vi "DOE Water Temperature Pressure.vi"(5 "Water Pressure":dbl, 6 "Data Logger Type":T1=enum."Agilent", 7 "Water Temperature":dbl, 8 "Error In":errorcluster, 9 "Output Array":dbl[](array[numeric]), 10 "TC Coefficients":T2, 11 "Kitchen Cluster in":T3) -> (0 "Error Out":errorcluster, 3 "Kitchen Cluster out":T3, 4 "sorted array":i32[](array[numeric]))   [LabVIEW 2016]
uses:
  Type Definitions/DOE Kitchen Control.ctl
  Utility/Type Definitions/UTILITY TC Coefficients.ctl
  Type Definitions/DOE Data Logger Type.ctl
  Utility/Type Definitions/UTILITY TC Coefficients Selector.ctl
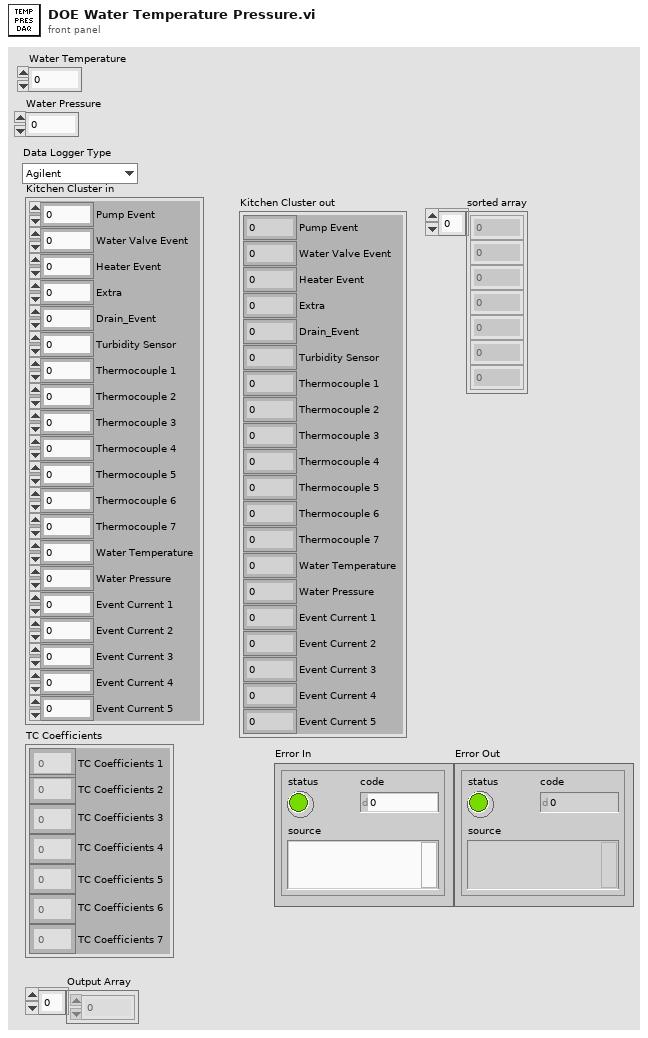
[diagram p1: front panel]
types:
  T1 = typedef "DOE Data Logger Type.ctl" = enum16{"MW100", "Agilent", "Agilent_Laurel_DC_Clamp"}
  T2 = typedef "UTILITY TC Coefficients.ctl" = cluster{"TC Coefficients 1":dbl[], "TC Coefficients 2":dbl[], "TC Coefficients 3":dbl[], "TC Coefficients 4":dbl[], "TC Coefficients 5":dbl[], "TC Coefficients 6":dbl[], "TC Coefficients 7":dbl[]}
  T3 = typedef "DOE Kitchen Control.ctl" = cluster{"Drain_Event":i16, "Pump Event":i16, "Water Valve Event":i16, "Heater Event":i16, "Extra":i16, "Turbidity Sensor":dbl, "Thermocouple 1":dbl, "Thermocouple 2":dbl, "Thermocouple 3":dbl, "Thermocouple 4":dbl, "Thermocouple 5":dbl, "Thermocouple 6":dbl, "Water Temperature":dbl, "Water Pressure":dbl, "Event Current 1":dbl, "Event Current 2":dbl, "Event Current 3":dbl, "Event Current 4":dbl, "Event Current 5":dbl, "Thermocouple 7":dbl}
  T4 = typedef "UTILITY TC Coefficients Selector.ctl" = enum16{"TC1", "TC2", "TC3", "TC4", "TC5", "TC6", "TC7"}
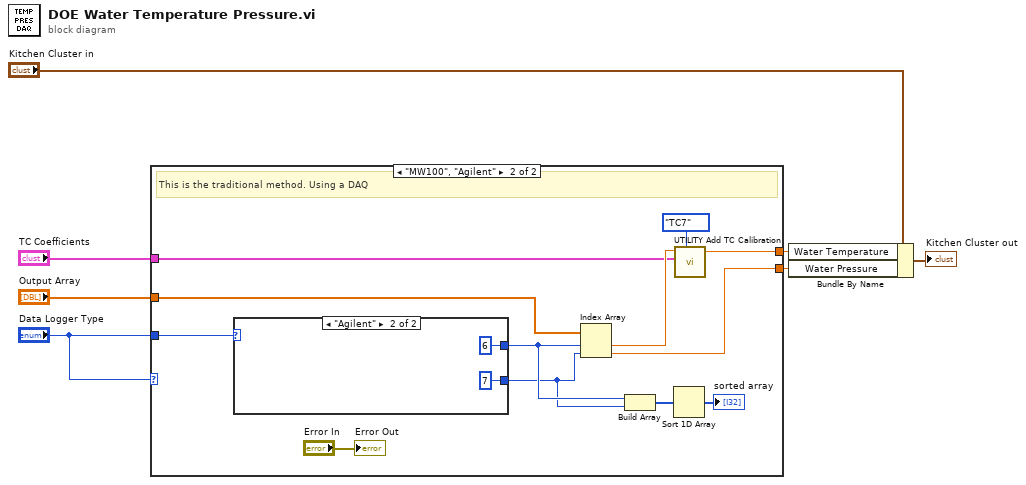
[diagram p0: block diagram]
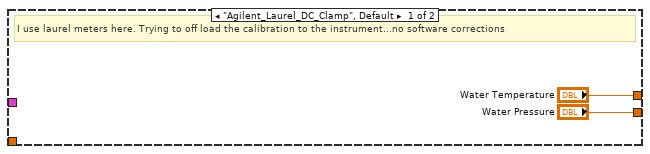
[diagram p2: hidden frame]
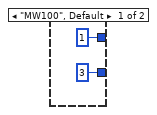
[diagram p3: hidden frame]
diagram:
  n1 = case shown="\"MW100\", \"Agilent\"" "Data Logger Type" {
    tunnel: ["Water Pressure" w21] -> w6
    tunnel: "Output Array" -> [_ w19]
    tunnel: ["Water Temperature" w18] -> w4
    tunnel: "TC Coefficients" -> [_ w17]
    tunnel: "Data Logger Type" -> [_ w14]
    frame "Agilent_Laurel_DC_Clamp", Default {
      # "I use laurel meters here. Trying to off load the calibration to the instrument...no software corrections"
    }
    frame "MW100", "Agilent" {
      # "This is the traditional method. Using a DAQ"
      n2 = case shown="\"Agilent\"" w14 {
        tunnel: [1 ("index") 6 ("index")] -> w13
        tunnel: [3 ("index") 7 ("index")] -> w12
        frame "MW100", Default {
        }
        frame "Agilent" {
        }
      }
      n3 = Index Array(array=w19, index #1=w13, index #2=w12) -> (element #1=w20:dbl, element #2=w21:dbl)
      n4 = Build Array(w13, w12) -> (w11:i32[])
      n5 = Sort 1D Array(array=w11) -> (sorted array=→"sorted array":i32[])
      n6 = call "UTILITY Add TC Calibration.vi"("Enum"=UTILITY_TC_Coefficients_Selector."TC7", "TC Coefficients"=w17, "Non Cal Temp"=w20) -> ("Calibrated Temp"=w18:dbl)  [unwired: 8 in]
      "Error Out" <- "Error In"
    }
  }
  n7 = Bundle By Name(cluster="Kitchen Cluster in", "Water Temperature"=w4, "Water Pressure"=w6) -> (→"Kitchen Cluster out":T3)
